vi "FSK_AddSync.vi"(8 "error in (no error)":errorcluster caption="错误输入（无错误）", 10 "code":dbl[](array[numeric]), 11 "PathIn":path) -> (0 "error out":errorcluster caption="错误输出", 2 "data":dbl[](array[numeric]) format="%#_13g", 3 "PathOut":path)   [LabVIEW 2015]
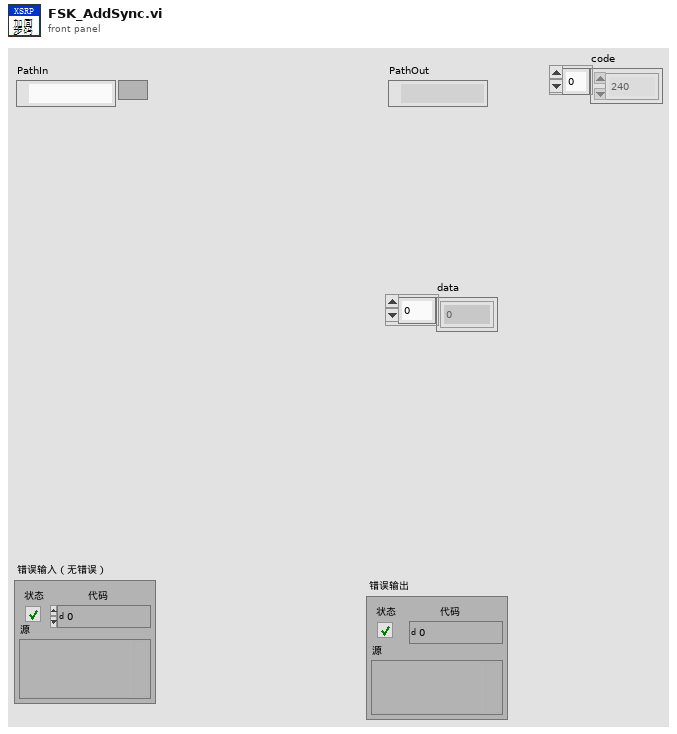
[diagram p1: front panel]
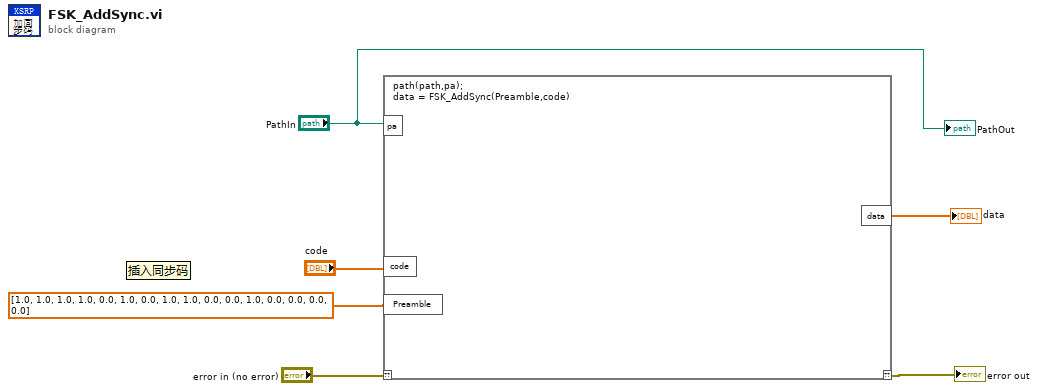
[diagram p0: block diagram]
diagram:
  n1 = script code="path(path,pa);\ndata = FSK_AddSync(Preamble,code)"("??"="error in (no error)", "pa"="PathIn", "code"="code", "Preamble"=dbl[] [1.0, 1.0, 1.0, 1.0, 0.0, 1.0, 0.0, 1.0, 1.0, 0.0, 0.0, 1.0, 0.0, 0.0, 0.0, 0.0] ("数组")) -> ("??"=→"error out":errorcluster, "data"=→"data":dbl[])
  "PathOut" <- "PathIn"
